vi "alarm map.vi"(8 "error in (no error)":errorcluster, 11 "map in":T2) -> (0 "error out":errorcluster, 2 "change?":bool, 3 "map out":T1)   [LabVIEW 2016, in "opSignIn.lvlib"]
uses:
  opSignIn.lvlib
  map in.ctl
  map out.ctl
  <vilib>/xml/Load XML File.vi
  <vilib>/xml/Close Reference(Node).vi
  <vilib>/xml/NI_XML.lvlib
  <resource>/objmgr/DOMUserDefRef.rc
panel:
  out "XML":string
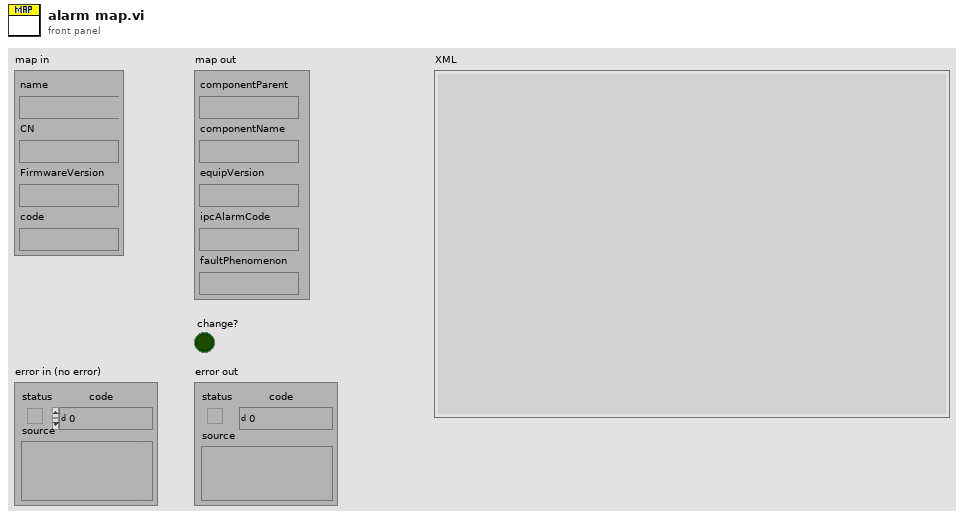
[diagram p1: front panel]
types:
  T1 = typedef "opSignIn.lvlib/map out.ctl" = cluster{"componentParent":string, "componentName":string, "equipVersion":string, "ipcAlarmCode":string, "faultPhenomenon":string}
  T2 = typedef "opSignIn.lvlib/map in.ctl" = cluster{"name":string, "CN":string, "FirmwareVersion":string, "code":string}
  T3 = cluster{"name":bool, "CN":bool, "FirmwareVersion":bool, "code":bool}
  T4 = cluster{"[0]":string, "[1]":string, "[2]":string, "[3]":string, "[4]":string}
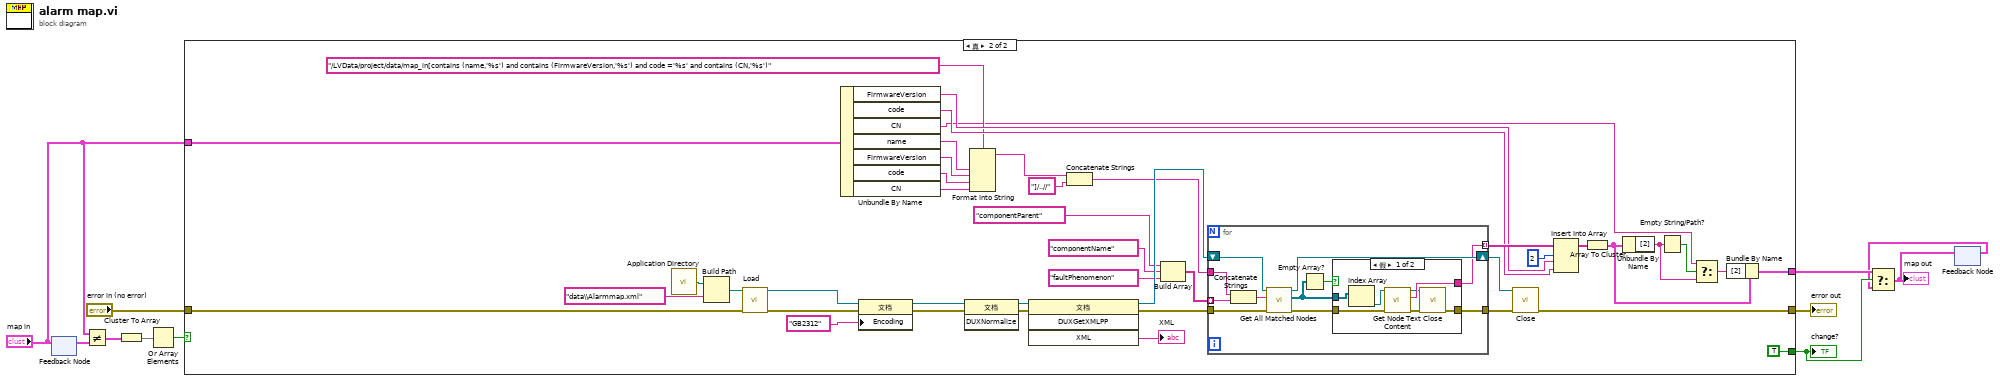
[diagram p0: block diagram]
diagram:
  n1 = feedback-in #1("map in") -> ()
  n2 = feedback #1() -> (w8:T2)  [unwired: 1 in]
  n3 = Not Equal?(x="map in", y=w8) -> (x != y?=w7:T3)
  n4 = Cluster To Array(cluster=w7) -> (array=w6:bool[])
  n5 = Or Array Elements(Boolean array=w6) -> (logical OR=w5:bool)
  n6 = case shown="真" w5 {
    tunnel: [_ w13] -> w3
    tunnel: [_ w53] -> w11
    tunnel: "error in (no error)" -> [_ w52]
    tunnel: "map in" -> [_ w51]
    tunnel: [_ TRUE] -> w4
    frame False {
    }
    frame True {
      n7 = call <vilib>:"Application Directory.vi"() -> ("Application Directory"=w37:path)
      n8 = Build Path(base path=w37, name or relative path="data\\Alarmmap.xml" ("字符串")) -> (appended path=w35:path)
      n9 = call-poly <vilib>:"Load.vi"("path to XML document"=w35, "error in (no error)"=w52) -> ("DOM document out"=w47:refnum<k20>, "error out"=w46:errorcluster)  [unwired: 11 in, 1 out]
      n10 = Unbundle By Name(w51) -> ("FirmwareVersion"=w23:string, "code"=w22:string, "CN"=w15:string, "name"=w29:string, "FirmwareVersion"=w38:string, "code"=w24:string, "CN"=w20:string)
      n11 = property on="属性节点" class="文档"(reference=w47, error in=w46, "Encoding"="GB2312" ("文档编码")) -> (reference out=w49:refnum<k20>, error out=w48:errorcluster)
      n12 = invoke on="调用节点" class="文档" method="DUXNormalize"(reference=w49, error in=w48) -> (reference out=w45:refnum<k20>, error out=w44:errorcluster)  [unwired: 1 in, 1 out]
      n13 = Format Into String(format string="/LVData/project/data/map_in[contains (name,'%s') and contains (FirmwareVersion,'%s') and code ='%s' and contains (CN,'%s')" ("字符串"), w29, w38, w24, w20) -> (resulting string=w34:string)  [unwired: 2 in, 1 out]
      n14 = invoke on="调用节点" class="文档" method="DUXGetXMLPP"(reference=w45, error in=w44) -> (reference out=w43:refnum<k20>, error out=w39:errorcluster, "XML"=→"XML":string)  [unwired: 2 in, 1 out]
      n15 = Concatenate Strings(w34, "]/..//" ("字符串")) -> (w40:string)
      n16 = Build Array("componentParent", "componentName", "faultPhenomenon") -> (w42:string[])
      n17 = for {
        tunnel: w40 -> [w61]
        tunnel: w42 -> [w60] mode=indexing
        tunnel: [w54] -> w26 mode=indexing
        tunnel: [w57] -> w31
        tunnel: w39 -> [w59]
        shift-right: [w63] -> w32
        shift-left: w43 -> [w64]
        n18 = Concatenate Strings(w61, w60) -> (w58:string)
        n19 = call <vilib>:"Get All Matched Nodes.vi"("error in (no error)"=w59, "XPath expression"=w58, "node in"=w64) -> ("error out"=w62:errorcluster, "node result array"=w55:refnum<k20>[], "node out"=w63:refnum<k20>)  [unwired: 6 in]
        n20 = Empty Array?(array=w55) -> (empty?=w56:bool)
        n21 = case shown="假" w56 {
          tunnel: [w71 _] -> w54
          tunnel: w62 -> [w70 w72]
          tunnel: [w67 w72] -> w57
          tunnel: w55 -> [w66 _]
          frame False {
            n22 = Index Array(array=w66) -> (element=w65:refnum<k20>)  [unwired: 1 in]
            n23 = call <vilib>:"Get Node Text Content.vi"("error in (no error)"=w70, "node in"=w65) -> ("error out"=w68:errorcluster, "node text"=w71:string, "node out"=w69:refnum<k20>)  [unwired: 7 in]
            n24 = call-poly <vilib>:"Close.vi"("error in (no error)"=w68, "node"=w69) -> ("error out"=w67:errorcluster)  [unwired: 7 out]
          }
          frame True {
          }
        }
      }
      n25 = call-poly <vilib>:"Close.vi"("error in (no error)"=w31, "node"=w32) -> ("error out"=w53:errorcluster)  [unwired: 7 out]
      n26 = Insert Into Array(array=w26, index=2 ("索引"), new element #1=w23, new element #2=w22) -> (w27:string[])
      n27 = Array To Cluster(array=w27) -> (cluster=w17:T4)
      n28 = Unbundle By Name(w17) -> ("[2]"=w14:string)
      n29 = Empty String/Path?(string/path=w14) -> (empty?=w16:bool)
      n30 = Select(t=w15, s=w16, f=w14) -> (s? t:f=w12:string)
      n31 = Bundle By Name(cluster=w17, "[2]"=w12) -> (w13:T4)
    }
  }
  "error out" <- w11
  "change?" <- w4
  n32 = feedback #2() -> (w1:T4)  [unwired: 1 in]
  n33 = Select(t=w3, s=w4, f=w1) -> (s? t:f=w2:T4)
  "map out" <- w2
  n34 = feedback-in #2(w2) -> ()
